vi "OdometrySubscriber.vi"(1 "error in":errorcluster) -> (0 "error out":errorcluster)   [LabVIEW 2014]
doc: "Reads in the odometry from the Turtlebot"
uses:
  <vilib>/Tufts CEEO ROS for LabVIEW Software/ROS/Code/Console/Servers/ServerSubs/TopicDef.ctl
  <vilib>/Tufts CEEO ROS for LabVIEW Software/ROS/Code/SubVIs/_ROSDirection.ctl
panel:
  out "2D Pose":cluster{"x":dbl, "y":dbl}
  out "Position Plot":cluster{"X":dbl, "Y":dbl}[](graph)
  out "Husky EKF Odometry":T1
  in  "Stop Subscribing":bool
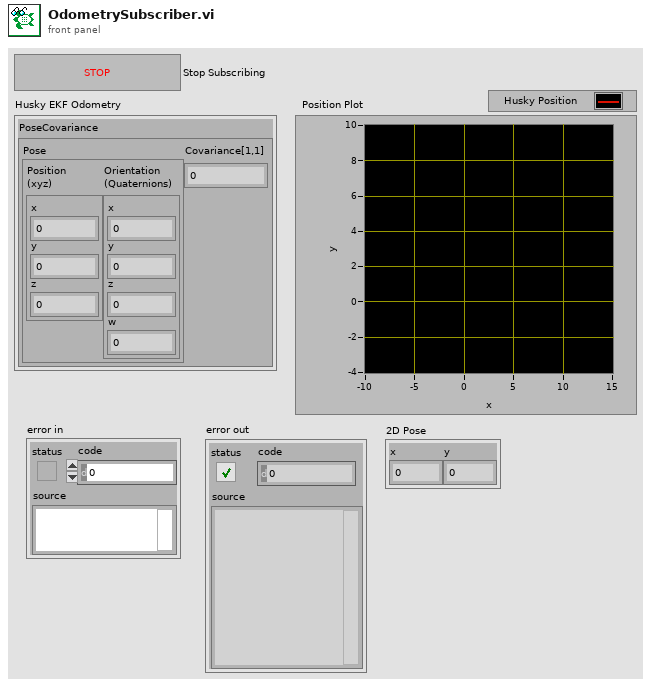
[diagram p1: front panel]
types:
  T1 = cluster{"PoseCovariance":cluster{"Pose":cluster{"Position\n(xyz)":cluster{"x":dbl, "y":dbl, "z":dbl}, "Orientation\n(Quaternions)":cluster{"x":dbl, "y":dbl, "z":dbl, "w":dbl}}, "Covariance[1,1]":dbl}}
  T2 = typedef "TopicDef.ctl" = cluster{"Topic":string, "Type":string, "Action":T3, "Update (ms)":u16, "queue size":u16}
  T3 = typedef "_ROSDirection.ctl" = enum16{"Node", "Publisher", "Subscriber", "ServiceClient", "ServiceProvider"}
  T4 = typedef "_ROSControl.ctl" = cluster{"topic port":u16, "Node":string, "topic":string, "type":string, "node port":u16, "error ":errorcluster, "Direction":T3, "Update (ms)":u16, "FIFO size":u16}
  T5 = cluster{"PoseCovariance":cluster{"Pose":cluster{"Point":cluster{"x":dbl, "y":dbl, "z":dbl}, "Quaternion":cluster{"x":dbl, "y":dbl, "z":dbl, "w":dbl}}, "Covariance":dbl}}
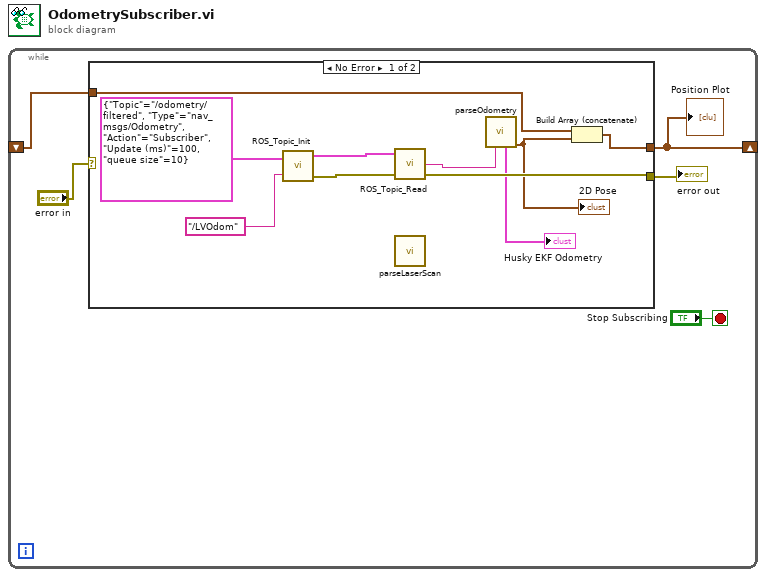
[diagram p0: block diagram]
diagram:
  n1 = while {
    shift-right: [w1] -> _
    shift-left: _ -> [w2]
    stop <- "Stop Subscribing" stop-if-true
    n2 = case shown="No Error" "error in" {
      selector: "error in" -> [_ w17]
      tunnel: [w11 w17] -> w5
      tunnel: w2 -> [w8 w16]
      tunnel: [w7 w16] -> w1
      frame No Error {
        n3 = call <vilib>:"ROS_Topic_Init.vi"("Definitions"=T2 {"Topic"="/odometry/filtered", "Type"="nav_msgs/Odometry", "Action"=enum."Subscriber", "Update (ms)"=100, "queue size"=10}, "node"="/LVOdom") -> ("ROS out"=w14:T4, "error out"=w13:errorcluster)  [unwired: 1 in]
        n4 = call <vilib>:"ROS_Topic_Read.vi"("error in (no error)"=w13, "ROS in"=w14) -> ("error out"=w11:errorcluster, "Reply"=w10:string)  [unwired: 1 in, 1 out]
        n5 = call "parseLaserScan.vi"() -> ()  [unwired: 4 in, 4 out]
        n6 = call "parseOdometry.vi"("msg in"=w10) -> ("Odometry"=→"Husky EKF Odometry":T5, "Pose 2D"=w6:cluster{"x":dbl, "y":dbl})  [unwired: 3 in, 3 out]
        "2D Pose" <- w6
        n7 = Build Array (concatenate)(w8, w6) -> (w7:cluster{"x":dbl, "y":dbl}[])
      }
      frame Error {
      }
    }
    "error out" <- w5
    "Position Plot" <- w1
  }
